vi "LecroySet.vi"(8 "error in":errorcluster) -> (0 "error out":errorcluster, 2 "Test Waveorm":dbl[](graph), 3 "VISA resource name out":refnum<visa-resource-name>)   [LabVIEW 2022 SP3]
uses:
  GaGe/-GageUtils/GageGlobals.vi
  <instrlib>/LeCroy Wave Series/LeCroy Wave Series.lvlib
panel:
  in  "Sampling Rate":u16(ring)=2 items=["50 MS/s", "100 MS/s", "250 MS/s"]
  # "Call this VI to load proper delay and ensure correct number of RF pts are acquired. User must set trigger levels, turn on channels, and set voltage scales for each channel."
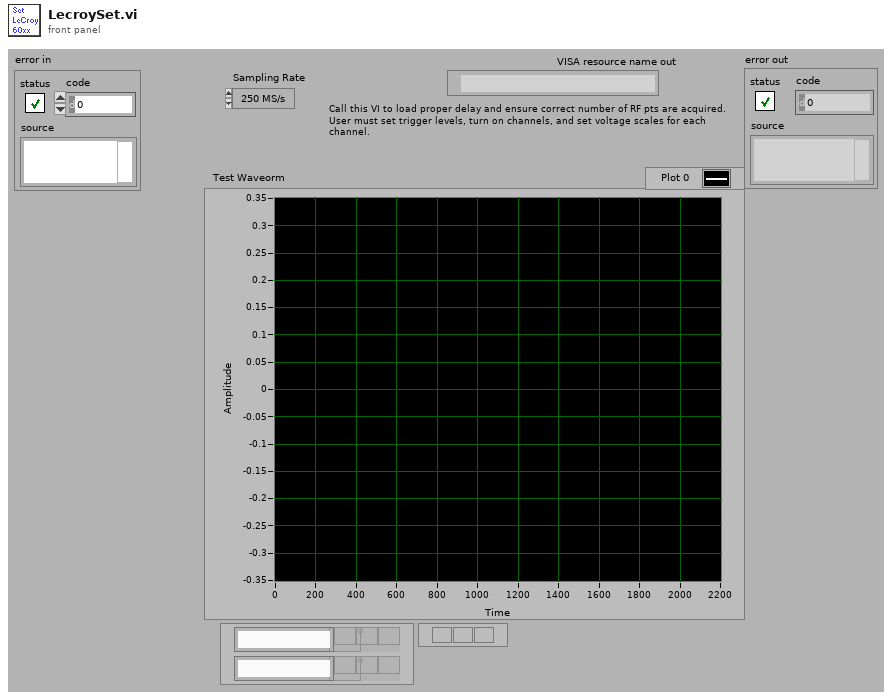
[diagram p1: front panel]
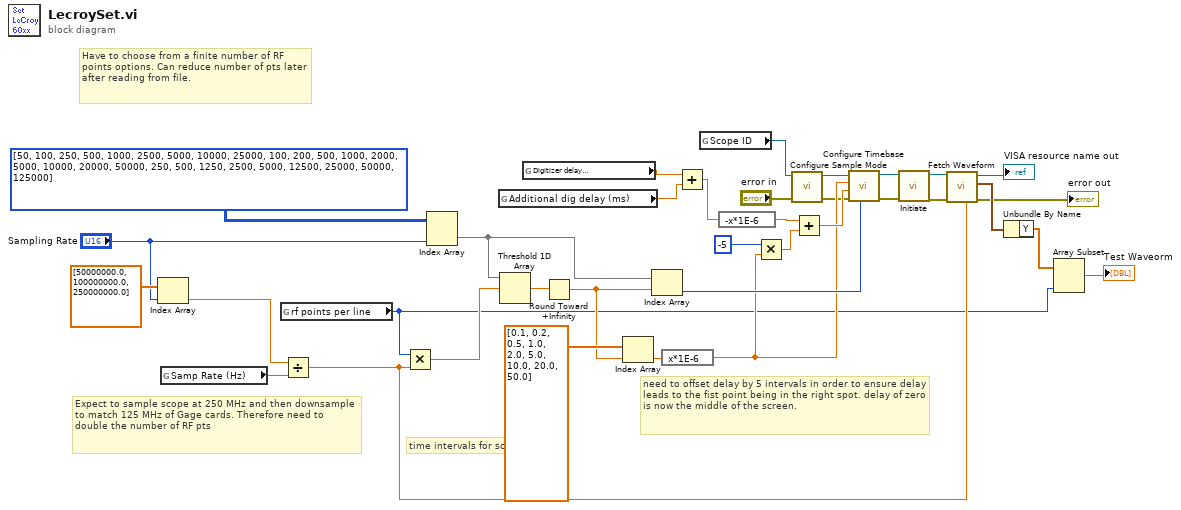
[diagram p0: block diagram]
diagram:
  # "time intervals for scope"
  # "need to offset delay by 5 intervals in order to ensure delay leads to the fist point being in the right spot. delay of zero is now the middle of the screen."
  # "Expect to sample scope at 250 MHz and then downsample to match 125 MHz of Gage cards. Therefore need to double the number of RF pts"
  # "Have to choose from a finite number of RF points options. Can reduce number of pts later after reading from file."
  n1 = Index Array(array=dbl[] [50000000.0, 100000000.0, 250000000.0], index="Sampling Rate") -> (element=w20:dbl)
  n2 = global read "GageGlobals.vi" "Samp Rate (Hz)"() -> (w22:dbl)
  n3 = global read "GageGlobals.vi" "rf points per line"() -> (w8:i32)
  n4 = Divide(x=w20, y=w22) -> (x/y=w10:dbl)
  n5 = Multiply(x=w8, y=w10) -> (x*y=w18:dbl)
  n6 = Index Array(array=i32[][] [[50, 100, 250, 500, 1000, 2500, 5000, 10000, 25000], [100, 200, 500, 1000, 2000, 5000, 10000, 20000, 50000], [250, 500, 1250, 2500, 5000, 12500, 25000, 50000, 125000]], index (row)="Sampling Rate") -> (element=w28:i32[])  [unwired: 1 in]
  n7 = global read "GageGlobals.vi" "Additional dig delay (ms)"() -> (w34:dbl)
  n8 = Threshold 1D Array(2:w18, 3:w28) -> (0:w30:dbl)  [unwired: 1 out]
  n9 = global read "GageGlobals.vi" "Digitizer delay\n (ms)"() -> (w35:dbl)
  n10 = Round Toward +Infinity(x=w30) -> (ceil(x): smallest int >= x=w25:dbl)
  n11 = Index Array(array=dbl[] [0.1, 0.2, 0.5, 1.0, 2.0, 5.0, 10.0, 20.0, 50.0], index=w25) -> (element=w26:dbl)
  n12 = Index Array(array=w28, index=w25) -> (element=w16:i32)
  n13 = expression code="x*1E-6"(w26) -> (w11:dbl)
  n14 = Add(x=w35, y=w34) -> (x+y=w33:dbl)
  n15 = global read "GageGlobals.vi" "Scope ID"() -> (w1:refnum<visa-resource-name>)
  n16 = expression code="-x*1E-6"(w33) -> (w13:dbl)
  n17 = Multiply(x=-5, y=w11) -> (x*y=w14:dbl)
  n18 = call <instrlib>:"Configure Sample Mode.vi"("error in (no error)"="error in", "VISA resource name"=w1) -> ("error out"=w3:errorcluster, "VISA resource name out"=w4:refnum<visa-resource-name>)  [unwired: 2 in, 6 out]
  n19 = Add(x=w13, y=w14) -> (x+y=w12:dbl)
  n20 = call <instrlib>:"Configure Timebase.vi"("Maximum Sample Points (500)"=w16, "error in (no error)"=w3, "Position (0.0 s)"=w12, "Timebase (0.0005 s)"=w11, "VISA resource name"=w4) -> ("error out"=w23:errorcluster, "VISA resource name out"=w24:refnum<visa-resource-name>)  [unwired: 5 out]
  n21 = call <instrlib>:"Initiate.vi"("error in (no error)"=w23, "VISA resource name"=w24) -> ("error out"=w31:errorcluster, "VISA resource name out"=w32:refnum<visa-resource-name>)  [unwired: 1 in, 7 out]
  n22 = call <instrlib>:"Fetch Waveform.vi"("Sparsing (0: Every point)"=w10, "error in (no error)"=w31, "VISA resource name"=w32) -> ("error out"=→"error out":errorcluster, "Waveform Graph"=w17:waveform(dbl), "VISA resource name out"=→"VISA resource name out":refnum<visa-resource-name>)  [unwired: 6 in]
  n23 = Unbundle By Name(w17) -> ("Y"=w9:dbl[])
  n24 = Array Subset(array=w9, length=w8) -> (→"Test Waveorm":dbl[])  [unwired: 1 in]
